vi "ZPL Config Program Data.vi"(6 "Settle (1 mS)":u32=1, 7 "Triggering value (for fix)":dbl, 8 "error":errorcluster, 9 "DATA":T1={"Value string"="", "Time string"="", "step"=0, "Counter"=1.0} {"Counter" min=1.0 max=65534.0 step=1.0; "step" items=["ONCE", "AUTO"]}, 10 "MODE":T2 {"init:cont" items=["0", "1"]; "Mode" items=["VOLTAGE", "CURRENT"]; "Progr Mode" items=["NONE", "FIX", "LIST", "WAVE"]}, 11 "VISA":refnum<visa-resource-name>="0") -> (0 "error out":errorcluster, 2 "final string":string, 3 "VISA out":refnum<visa-resource-name>="0")   [LabVIEW 2015]
doc: "This VI sets the advance waveform. There are four modes \nNONE - is regular operation. \nFIX - In this mode of output control, each triggered output voltage or current value is explicitly specified by a triggered-level command (for example, VOLT:TRIG 20 or CURR:TRIG 1.55). The trigger then causes the output to change to this pending triggered level.\nLIST - This mode occurs when the VOLT:MODE LIST or CURR:MODE LIST command is programmed. In this mode of output operation, the triggered output voltage or current levels are specified within a list and the trigger controls the sequencing through the values in the list.\nWAVE -This mode occurs when the VOLT:MODE WAVE or CURR:MODE WAVE command is programmed. In this mode of output operation, the triggered output voltage or current levels and rise and fall slope are specified within a list and the trigger controls the sequencing through the values in the list.\n \nIf STEP AUTO has been programmed, the output automatically repeat waveforms when get only first trigger until it counting will be completed. \nIf STEP ONCE has been programmed, the output wait trigger before start repeat each waveform list. \n \nThis command sets the number of times that the list is executed before it is completed. The command accepts parameters in the range 1 through 9.9E37, but any number greater than 65534 is interpreted as INFinity. Use INF if you wish to execute a list indefinitely.\n\nIf INIT:CONT is OFF, then INIT enables the trigger subsystem only for a single trigger action. The subsystem must be enabled prior to each subsequent trigger action. If INIT:CONT is ON, then the trigger system is continuously enabled and INIT is redundant.\n\nThis VI will wait for \"Settle\" milliseconds after setting the limit to allow the output to reach the new setting. If unwired, there will be no delay"
panel:
  # "Lambda ZPLUS \n Serial Port\n  DC Power Supplies"
  # "Set the NONE, FIX, LIST, WAVE\n modes condition"
  # "for LIST and WAVE only"
  # "values V/A  Example :3,5.00,2.45"
  # "for LIST and WAVE only"
  # "values sec  Example :3,.2,0.003"
  # "for LIST and WAVE only"
  # "for LIST and WAVE only"
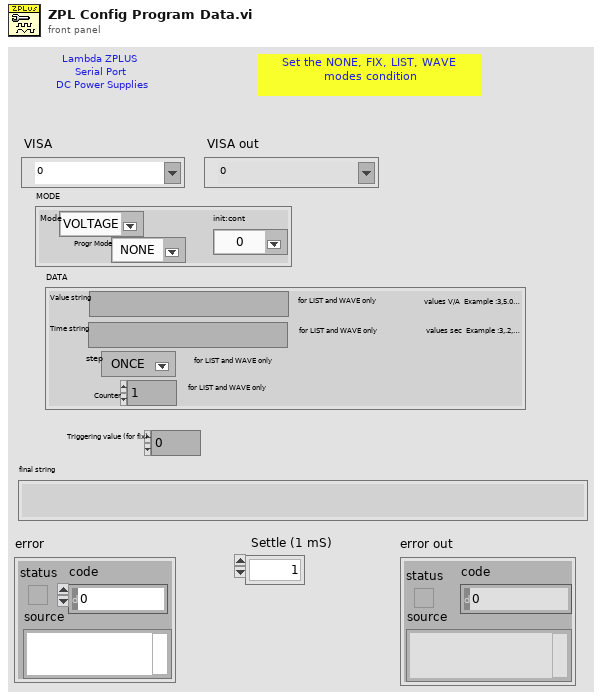
[diagram p1: front panel]
types:
  T1 = cluster{"Value string":string, "Time string":string, "step":u16, "Counter":dbl}
  T2 = cluster{"Progr Mode":u16, "Mode":u16, "init:cont":u16}
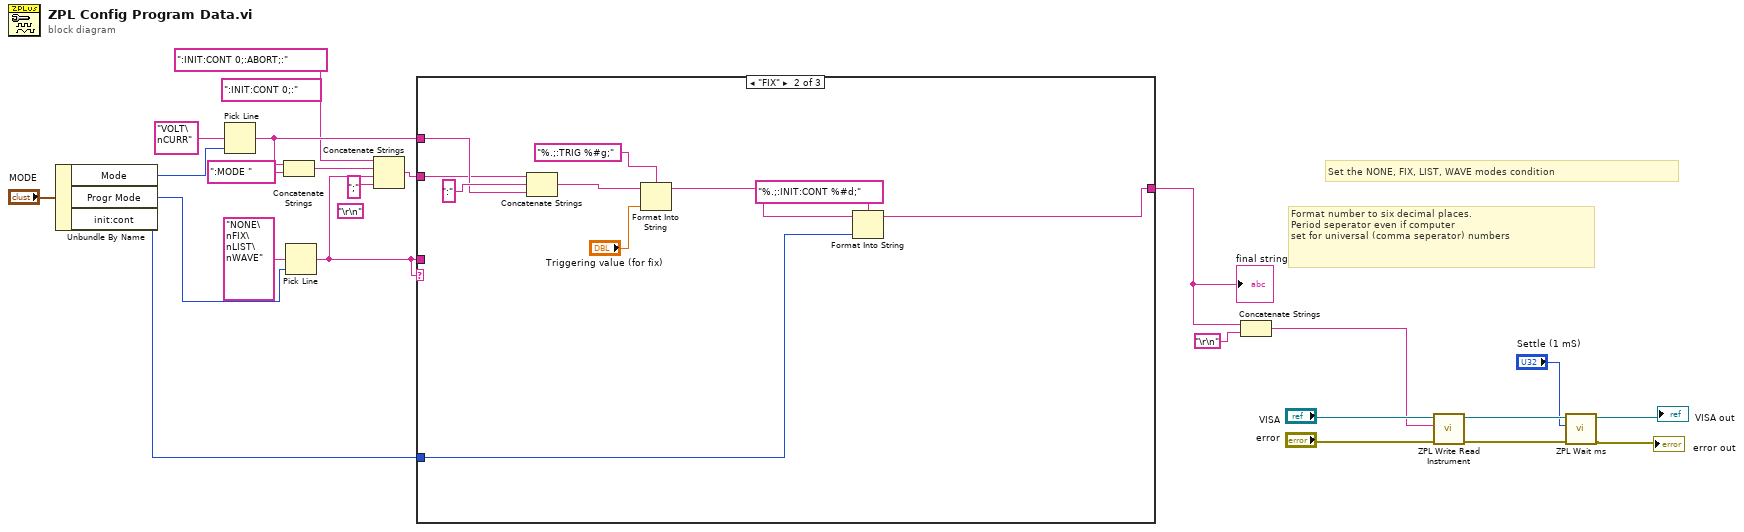
[diagram p0: block diagram]
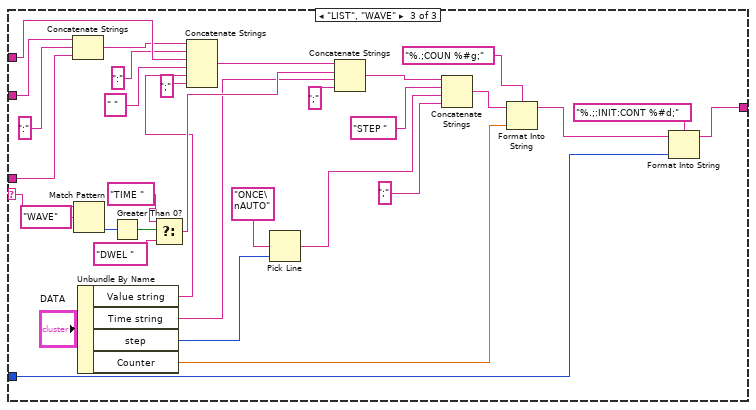
[diagram p3: hidden frame]
diagram:
  (unwired) ":INIT:CONT 0;:" ("Write Command/Query SCPI")
  (unwired) "\r\n"
  # "Format number to six decimal places.\nPeriod seperator even if computer \nset for universal (comma seperator) numbers"
  # "Set the NONE, FIX, LIST, WAVE modes condition"
  n1 = Unbundle By Name("MODE") -> ("Mode"=w6:u16, "Progr Mode"=w5:u16, "init:cont"=w4:u16)
  n2 = Pick Line(multi-line string="VOLT\nCURR" ("format string"), line index=w6) -> (output string=w11:string)  [unwired: 1 in]
  n3 = Concatenate Strings(w11, ":MODE " ("string")) -> (w13:string)
  n4 = Pick Line(multi-line string="NONE\nFIX\nLIST\nWAVE", line index=w5) -> (output string=w9:string)  [unwired: 1 in]
  n5 = Concatenate Strings(":INIT:CONT 0;:ABORT;:" ("Write Command/Query SCPI"), w13, w9, ";" ("string (\"\")")) -> (w10:string)
  n6 = case shown="\"FIX\"" w9 {
    selector: w9 -> [_ _ w52]
    tunnel: w11 -> [_ w33 w60]
    tunnel: [w24 w26 w38] -> w8
    tunnel: w10 -> [w24 w29 w35]
    tunnel: w9 -> [_ _ w57]
    tunnel: w4 -> [_ w27 w39]
    frame "NONE", Default {
    }
    frame "FIX" {
      n7 = Concatenate Strings(w29, ":" ("string"), w33) -> (w30:string)
      n8 = Format Into String(format string="%.;:TRIG %#g;", initial string=w30, "Triggering value (for fix)") -> (resulting string=w25:string)  [unwired: 1 in, 1 out]
      n9 = Format Into String(format string="%.;:INIT:CONT %#d;", initial string=w25, w27) -> (resulting string=w26:string)  [unwired: 1 in, 1 out]
    }
    frame "LIST", "WAVE" {
      n10 = Concatenate Strings(w35, ":" ("string"), w57) -> (w56:string)
      n11 = Match Pattern(string=w52, regular expression="WAVE") -> (offset past match=w53:i32)  [unwired: 1 in, 3 out]
      n12 = Unbundle By Name("DATA") -> ("Value string"=w43:string, "Time string"=w42:string, "step"=w44:u16, "Counter"=w41:dbl)
      n13 = Greater Than 0?(x=w53) -> (x > 0?=w50:bool)
      n14 = Select(t="TIME " ("string"), s=w50, f="DWEL " ("string")) -> (s? t:f=w48:string)
      n15 = Concatenate Strings(w56, ":" ("string"), w60, " " ("string"), w43, ";" ("string (\"\")")) -> (w62:string)
      n16 = Pick Line(multi-line string="ONCE\nAUTO" ("format string"), line index=w44) -> (output string=w47:string)  [unwired: 1 in]
      n17 = Concatenate Strings(w62, w48, w42, ";" ("string (\"\")")) -> (w61:string)
      n18 = Concatenate Strings(w61, "STEP " ("string"), w47, ";" ("string (\"\")")) -> (w58:string)
      n19 = Format Into String(format string="%.;COUN %#g;", initial string=w58, w41) -> (resulting string=w37:string)  [unwired: 1 in, 1 out]
      n20 = Format Into String(format string="%.;:INIT:CONT %#d;", initial string=w37, w39) -> (resulting string=w38:string)  [unwired: 1 in, 1 out]
    }
  }
  "final string" <- w8
  n21 = Concatenate Strings(w8, "\r\n") -> (w3:string)
  n22 = call "ZPL Write Read Instrument.vi"("error in"="error", "Write Command/Query SCPI"=w3, "VISA"="VISA") -> ("error out"=w20:errorcluster, "VISA  out"=w21:refnum<visa-resource-name>)  [unwired: 6 in, 1 out]
  n23 = call "ZPL Wait ms.vi"("error"=w20, "Delay (1 mS)"="Settle (1 mS)", "VISA"=w21) -> ("error out"=→"error out":errorcluster, "VISA out"=→"VISA out":refnum<visa-resource-name>)  [unwired: 7 in]
